vi "2_RGT_Table.vi"   [LabVIEW 2014]
uses:
  <vilib>/Utility/NIReport.llb/NI_report.lvclass
  <vilib>/Utility/NIReport.llb/Append Numeric Table to Report (wrap).vi
types:
  T1 = enum16{"Standard Report", "HTML", "Word", "Excel"}
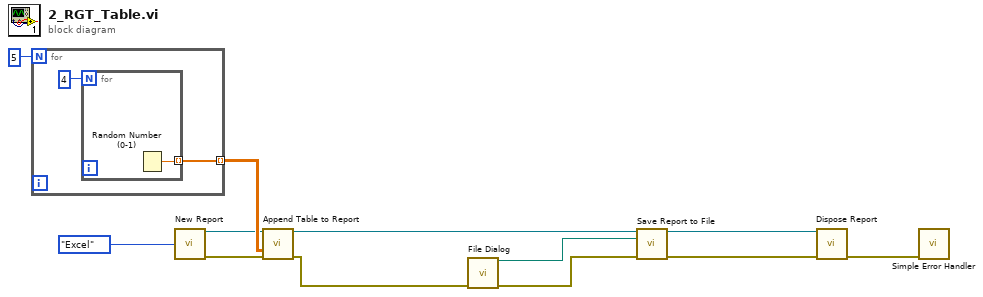
[diagram p0: block diagram]
diagram:
  n1 = for {
    N: 5 -> [_]
    tunnel: [w14] -> w11 mode=indexing
    n2 = for {
      N: 4 -> [_]
      tunnel: [w15] -> w14 mode=indexing
      n3 = Random Number (0-1)() -> (number: 0 to 1=w15:dbl)
    }
  }
  n4 = call <vilib>:"New Report.vi"("report type"=T1."Excel") -> ("report out"=w9:refnum<class "NI_report.lvclass">, "error out"=w8:errorcluster)  [unwired: 13 in]
  n5 = call-poly <vilib>:"Append Table to Report.vi"("report in"=w9, "numerical data"=w11, "error in (no error)"=w8) -> ("report out"=w2:refnum<class "NI_report.lvclass">, "error out"=w1:errorcluster)  [unwired: 9 in, 2 out]
  n6 = call "File Dialog"("error in"=w1) -> ("selected path"=w6:path, "error out"=w5:errorcluster)  [unwired: 11 in, 2 out]
  n7 = call-dynamic "Save Report to File.vi"("report in"=w2, "report file path"=w6, "error in (no error)"=w5) -> ("report out"=w4:refnum<class "NI_report.lvclass">, "error out"=w3:errorcluster)  [unwired: 11 in]
  n8 = call-dynamic "Dispose Report.vi"("report in"=w4, "error in (no error)"=w3) -> ("error out"=w7:errorcluster)  [unwired: 13 in]
  n9 = call <vilib>:"Simple Error Handler.vi"("error in (no error)"=w7) -> ()  [unwired: 4 in, 5 out]
